vi "shiftRegister.vi"() -> ()   [LabVIEW 2018]
panel:
  out "Numeric":i32
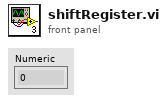
[diagram p1: front panel]
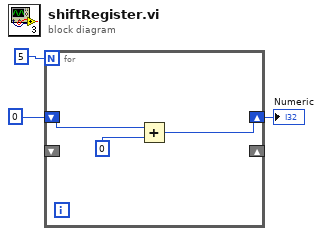
[diagram p0: block diagram]
diagram:
  n1 = for {
    N: 5 -> [_]
    shift-right: [w4] -> w1
    shift-left: 0 -> [w5]
    shift-right: _ -> [_]
    shift-left: _ -> [_]
    n2 = Add(x=w5, y=0) -> (x+y=w4:i32)
  }
  "Numeric" <- w1
